vi "Get Solenoid From Valve Enum.vi"(10 "Valve":T1) -> (0 "Use In Standby":bool, 2 "Port":u8)   [LabVIEW 2015]
uses:
  Valve Name Enum.ctl
  Valve Port Mapping Action.ctl
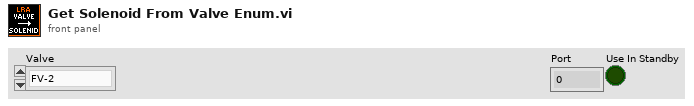
[diagram p1: front panel]
types:
  T1 = typedef "Valve Name Enum.ctl" = enum16{"FV-2", "FV-3", "FV-4", "OV-2", "OV-3", "OV-4", "NV-2", "COMP"}
  T2 = typedef "Valve Port Mapping Action.ctl" = enum16{"Get", "Set"}
  T3 = typedef "Valve Port Mapping.ctl" = cluster{"Valve":T1, "Port":u8, "Use In Standby":bool}
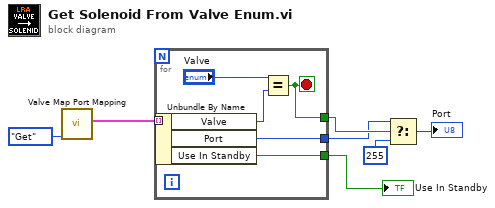
[diagram p0: block diagram]
diagram:
  n1 = call "Valve Map Port Mapping.vi"("Action"=Valve_Port_Mapping_Action."Get") -> ("Mapping List"=w6:T3[])  [unwired: 10 in]
  n2 = for {
    tunnel: w6 -> [w13] mode=indexing
    tunnel: [w10] -> w4
    tunnel: [w9] -> w5
    tunnel: [w8] -> w1
    stop <- w9 stop-if-true
    n3 = Unbundle By Name(w13) -> ("Valve"=w12:T1, "Port"=w10:u8, "Use In Standby"=w8:bool)
    n4 = Equal?(x="Valve", y=w12) -> (x = y?=w9:bool)
  }
  "Use In Standby" <- w1
  n5 = Select(t=w4, s=w5, f=u8 255) -> (s? t:f=→"Port":u8)
